vi "Build_Asylum_StopPISLoop.vi"(8 "error in (no error)":errorcluster, 11 "whichLoop":i32) -> (0 "error out":errorcluster, 3 "Command":string)   [LabVIEW 2016]
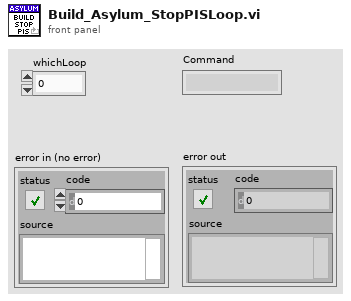
[diagram p1: front panel]
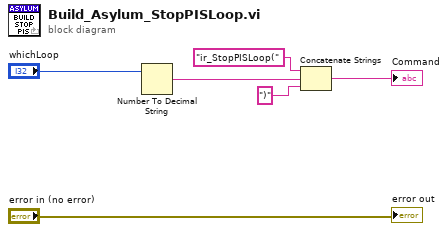
[diagram p0: block diagram]
diagram:
  n1 = Number To Decimal String(number="whichLoop") -> (decimal integer string=w4:string)  [unwired: 1 in]
  n2 = Concatenate Strings("ir_StopPISLoop(" ("string"), w4, ")" ("string")) -> (→"Command":string)
  "error out" <- "error in (no error)"
